vi "Write_File+_[U16].ph.vi"(6 "1D array":u16[](array[numeric]), 7 "2D array":u16[][](array[numeric]), 8 "error in (no error)":errorcluster, 9 "pos offset (bytes:0)":i32, 10 "pos mode (rel. to end:1)":enum16{"start", "end", "current"}(ring)=enum."end", 11 "refnum":refnum<file>) -> (0 "error out":errorcluster, 1 "mark after write (bytes)":i32, 3 "dup refnum":refnum<file>)   [LabVIEW 2010]
doc: "Writes a 2D or 1D array of signed word integers (I16) to a byte stream file at the specified location; the default location is at the end of file. The VI does incoming and internal error checking and does not write if an incoming error occurs.\n\nrefnum is the reference number of the open file.\n\npos mode specifies where the write begins relative to pos offset:\n\n 0: at the beginning of the file plus pos offset.\n\n 1: at the end of the file plus pos offset. This is the default value.\n\n 2: at the current file mark plus pos offset.\n\npos offset specifies in bytes how far from the location specified by pos mode that the operation begins. The default value is 0. Byte units rather than integer (2 byte) units for flexibility, for example, so that a file can contain a text header written with Write File+ (string) followed by arrays of number written with Write File+ [I16].\n\n2D array contains the signed word integers the VI writes to the file if 1D array is not wired or is empty.\n\n1D array contains signed word integers the VI writes to the file if this input is not empty.\n\nerror in is a cluster of three elements (error?, code, and source) that describe the upstream error state, that is, the existance of any error preceeding the execution of the VI. The VI executes normally only if no incoming error exists; otherwise it merely passes the error in value to error out. error? is TRUE if an error occurred; the default value is FALSE. code is the error code; the default value is 0. source is in most cases the name of the VI or function that produced the error; the default value is an empty string.\n\ndup refnum is a flow-though parameter with the same value as refnum.\n\nmark after write see above.\n\nerror out is a cluster of three elements (error?, code, and source) that describe the error state following the execution of the VI. If an incoming error does not exist, the VI executes normally and error out describes the VI's error state; if an incoming error exists, error out equals error in."
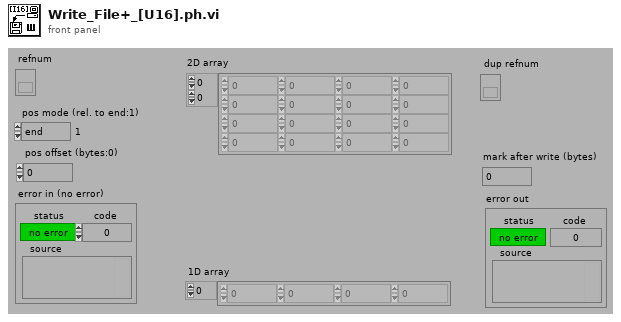
[diagram p1: front panel]
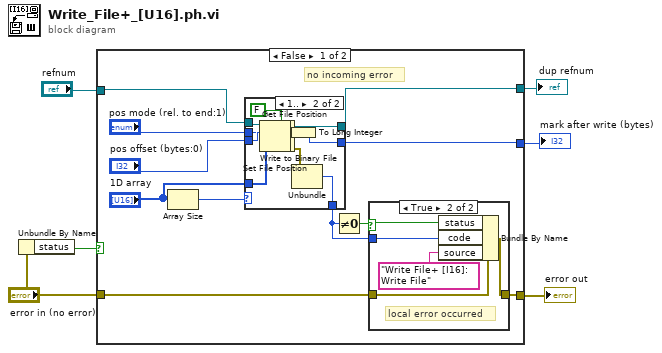
[diagram p0: block diagram]
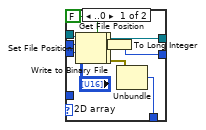
[diagram p3: hidden frame]
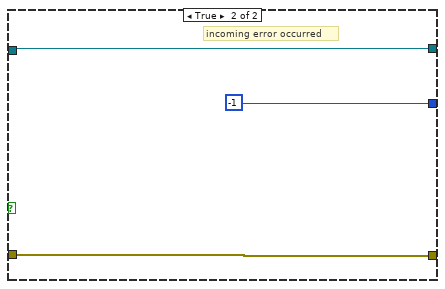
[diagram p4: hidden frame]
diagram:
  n1 = Unbundle By Name("error in (no error)") -> ("status"=w6:bool)
  n2 = case shown="False" w6 {
    tunnel: [w9 w53] -> w5
    tunnel: [w11 -1] -> w2
    tunnel: [w13 w52] -> w4
    tunnel: "refnum" -> [w14 w52]
    tunnel: "error in (no error)" -> [w10 w53]
    frame False {
      # "no incoming error"
      n3 = Array Size(array="1D array") -> (size(s)=w17:i32)
      n4 = case shown="1.." w17 {
        tunnel: "1D array" -> [_ w51]
        tunnel: "pos mode (rel. to end:1)" -> [w30 w44]
        tunnel: "pos offset (bytes:0)" -> [w36 w47]
        tunnel: w14 -> [w35 w48]
        tunnel: [w34 w50] -> w13
        tunnel: [w33 w49] -> w11
        tunnel: [w31 w46] -> w8
        frame ..0 {
          n5 = Set File Position(offset (in bytes) (0)=w36, refnum=w35, from (0:start)=w30) -> (refnum out=w29:refnum<file>, error out=w28:errorcluster)  [unwired: 1 in]
          n6 = Write to Binary File(file (use dialog)=w29, data="2D array", error in=w28, 5:FALSE ("prepend array or string size? (T)")) -> (refnum out=w27:refnum<file>, error out=w26:errorcluster)  [unwired: 3 out]
          n7 = Get File Position(4:w26, 7:w27) -> (0:w32:errorcluster, 2:w25:i64, 3:w34:refnum<file>)
          n8 = To Long Integer(number=w25) -> (32bit integer=w33:i32)
          n9 = Unbundle(w32) -> ("code"=w31:i32)  [unwired: 2 out]
        }
        frame 1.. {
          n10 = Set File Position(offset (in bytes) (0)=w47, refnum=w48, from (0:start)=w44) -> (refnum out=w43:refnum<file>, error out=w42:errorcluster)  [unwired: 1 in]
          n11 = Write to Binary File(file (use dialog)=w43, data=w51, error in=w42, 5:FALSE ("prepend array or string size? (T)")) -> (refnum out=w41:refnum<file>, error out=w40:errorcluster)  [unwired: 3 out]
          n12 = Get File Position(4:w40, 7:w41) -> (0:w45:errorcluster, 2:w39:i64, 3:w50:refnum<file>)
          n13 = To Long Integer(number=w39) -> (32bit integer=w49:i32)
          n14 = Unbundle(w45) -> ("code"=w46:i32)  [unwired: 2 out]
        }
      }
      n15 = Not Equal To 0?(x=w8) -> (x != 0?=w7:bool)
      n16 = case shown="True" w7 {
        selector: w7 -> [_ w19]
        tunnel: w8 -> [_ w22]
        tunnel: [w18 w23] -> w9
        tunnel: w10 -> [w18 w20]
        frame False {
          # "no local error"
        }
        frame True {
          # "local error occurred"
          n17 = Bundle By Name(cluster=w20, "status"=w19, "code"=w22, "source"="Write File+ [I16]: Write File") -> (w23:errorcluster)
        }
      }
    }
    frame True {
      # "incoming error occurred"
    }
  }
  "error out" <- w5
  "mark after write (bytes)" <- w2
  "dup refnum" <- w4
